vi "Web Service Authentication.vi"(8 "error in (no error)":errorcluster, 9 "Get/Set":enum16{"Get", "Set"}(ring), 11 "Web Service Authentication":T1) -> (0 "error out":errorcluster, 3 "Web Service Authentication 2":T1)   [LabVIEW 2017, in "WebServiceImporter.lvlib" / "ProxyDll Generator.lvlib"]
uses:
  <vilib>/Platform/WebService/ProxyDll Generator/ProxyDll Generator.lvlib
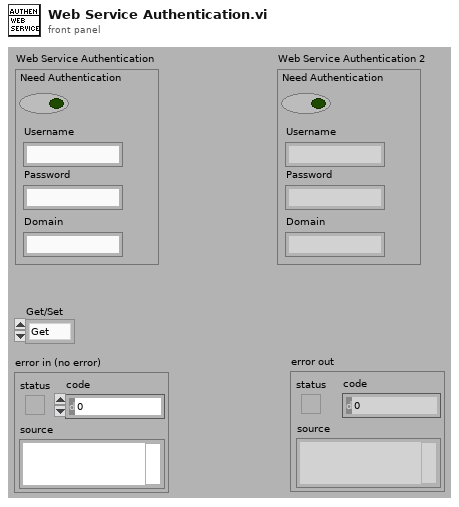
[diagram p1: front panel]
types:
  T1 = cluster{"Need Authentication":bool, "Username":string, "Password":string, "Domain":string}
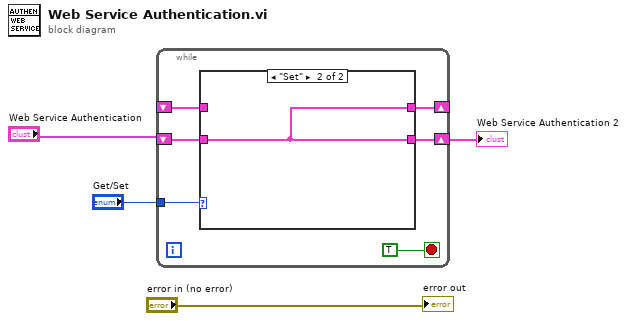
[diagram p0: block diagram]
diagram:
  n1 = while {
    tunnel: "Get/Set" -> [w9]
    shift-right: [w8] -> _
    shift-left: _ -> [w5]
    shift-right: [w7] -> w1
    shift-left: "Web Service Authentication" -> [w6]
    stop <- TRUE stop-if-true
    n2 = case shown="\"Set\"" w9 {
      tunnel: w5 -> [w11 _]
      tunnel: [w11 w12] -> w8
      tunnel: [w11 w12] -> w7
      tunnel: w6 -> [_ w12]
      frame "Get", Default {
      }
      frame "Set" {
      }
    }
  }
  "Web Service Authentication 2" <- w1
  "error out" <- "error in (no error)"
